vi "PID_controller_20.vi"() -> ()   [LabVIEW 2011]
panel:
  out "tFit_array":dbl[](array[numeric])
  out "PFit_array":dbl[](array[numeric])
  out "error array":dbl[](array[numeric])
  out "dt array":dbl[](array[numeric])
  out "Pset array":dbl[](array[numeric])
  out "t array":dbl[](array[numeric])
  out "P array":dbl[](array[numeric])
  in  "Local":bool
  in  "Hold":bool
  out "tune_Method":u16(ring) items=["Setpoint", "Angle"]
  in  "Method":u16(ring)=1 items=["Setpoint", "Angle"]
  in  "Setpoint":u16(ring)=2 items=["A", "B", "C", "D"]
  out "tuning":bool
  in  "Tune":bool
  out "Tune Set Point (torr)":dbl format="%.2f"
  in  "stop":bool
  out "err_avg":dbl
  out "Setpoint":string
  in  "Ks":dbl
  out "dt(s)":dbl
  out "windup error":dbl
  out "tPrev":dbl
  out "target value":dbl
  out "error":dbl
  out "tStart(s)":dbl
  out "S00":dbl
  out "S10":dbl
  out "S20":dbl
  out "S11":dbl
  out "S01":dbl
  out "weight array":dbl[](array[numeric])
  in  "# of points to watch":i32=60
  in  "tSmooth(s)":dbl=4.0
  out "IO error":errorcluster
  out "first":bool=TRUE
  out "XY Graph":cluster{"Value":dbl[], "Value":dbl[]}[](graph)
  out "current value":dbl
  in  "Period (s)":dbl=1.0
  out "dValue":dbl
  out "derivative":dbl
  out "integral":dbl
  in  "Angle (deg)":dbl format="%.1f"
  in  "Kd":dbl=0.4
  in  "Ki":dbl
  in  "Kp":dbl=0.1
  out "P (torr)":dbl format="%.2f"
  in  "Set Point (torr)":dbl format="%.2f"
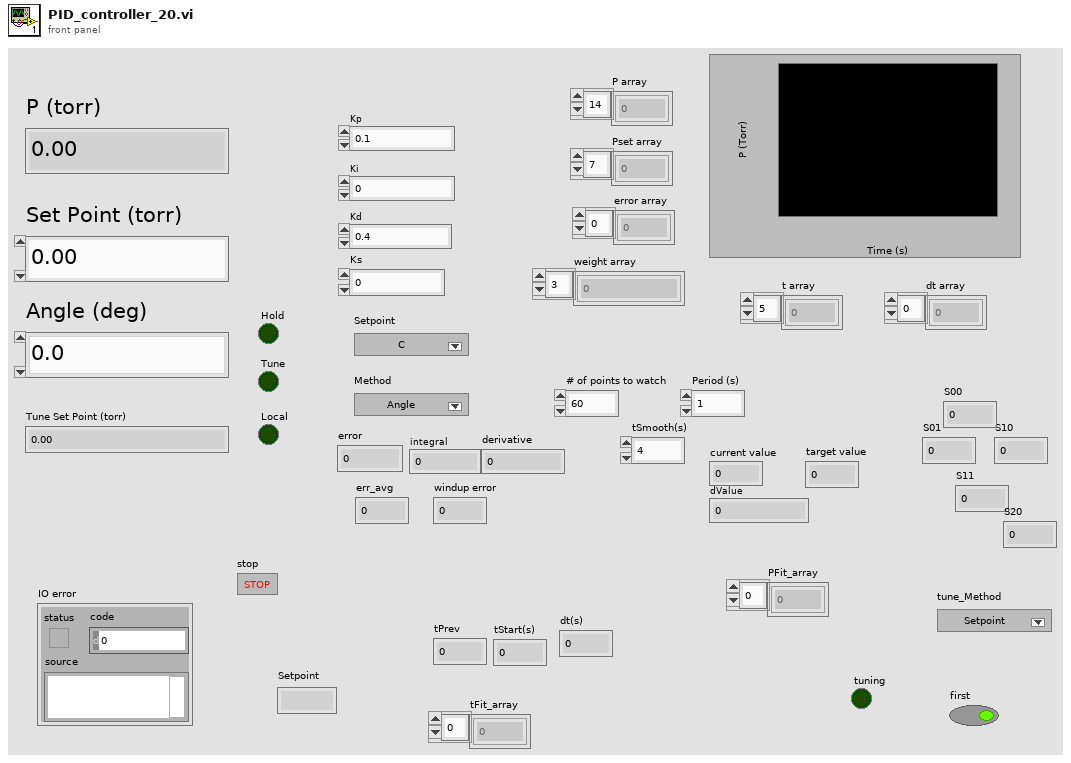
[diagram p1: front panel]
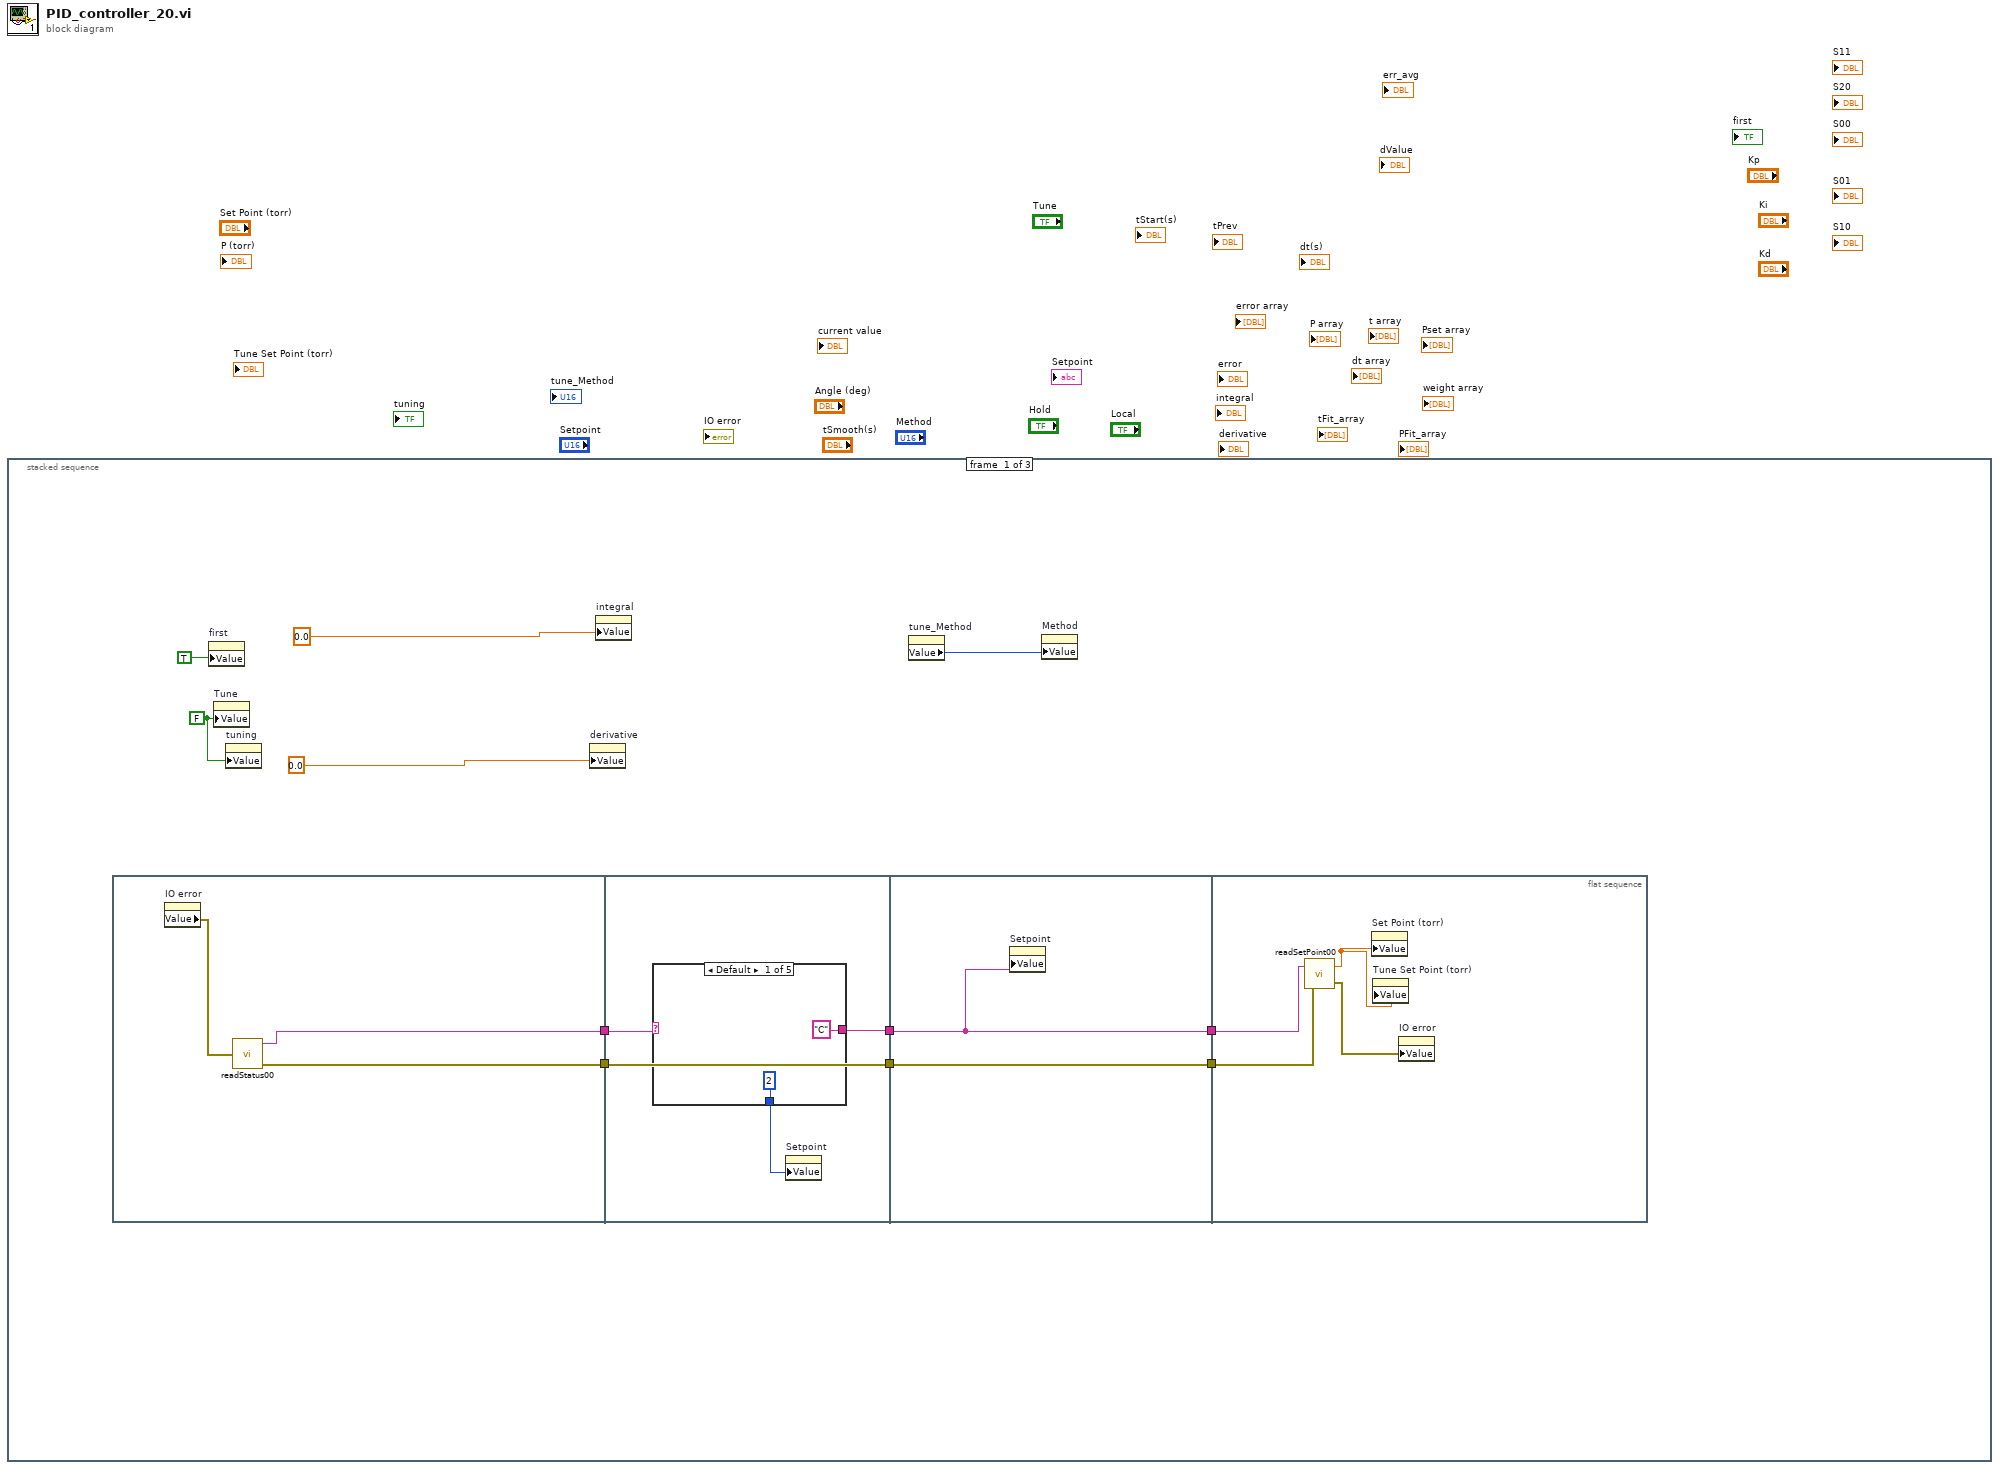
[diagram p0: block diagram]
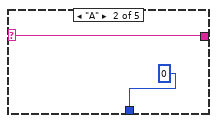
[diagram p2: hidden frame]
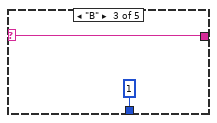
[diagram p3: hidden frame]
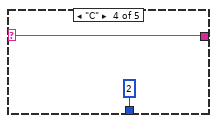
[diagram p4: hidden frame]
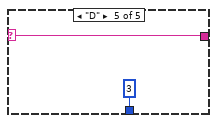
[diagram p5: hidden frame]
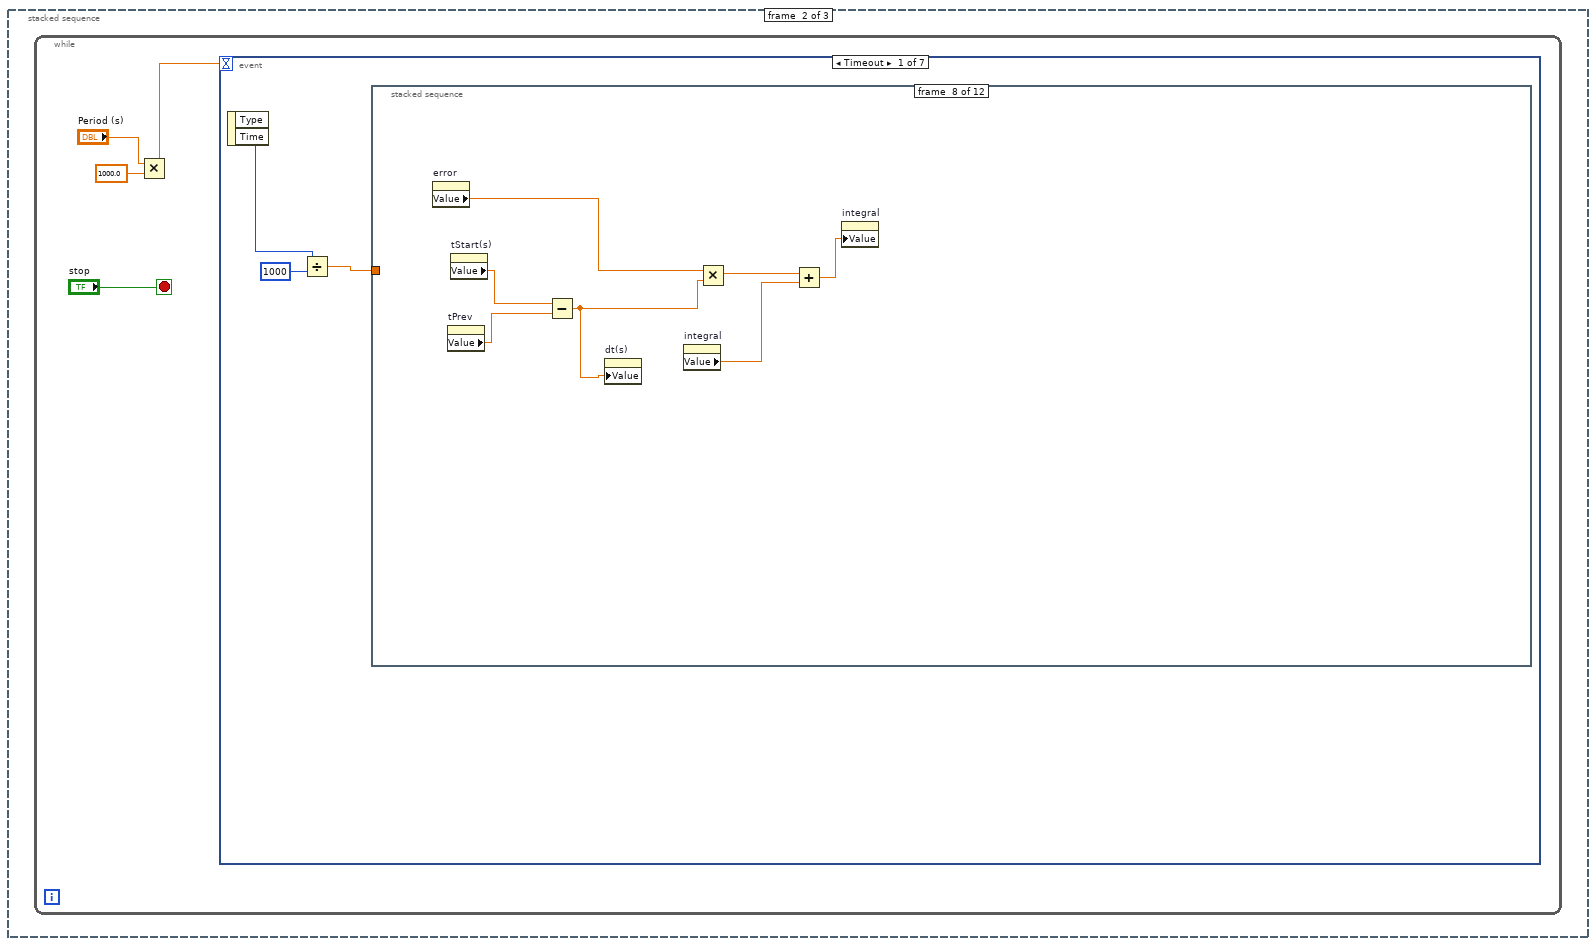
[diagram p6: hidden frame]
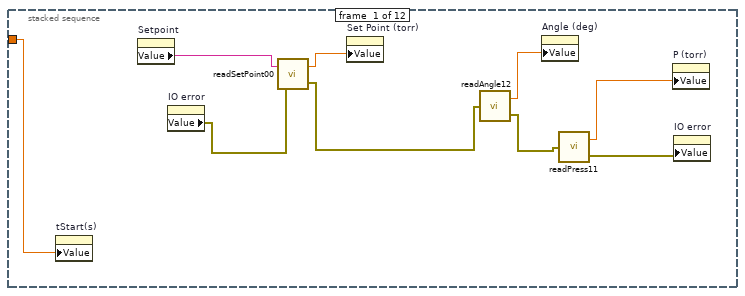
[diagram p7: hidden frame]
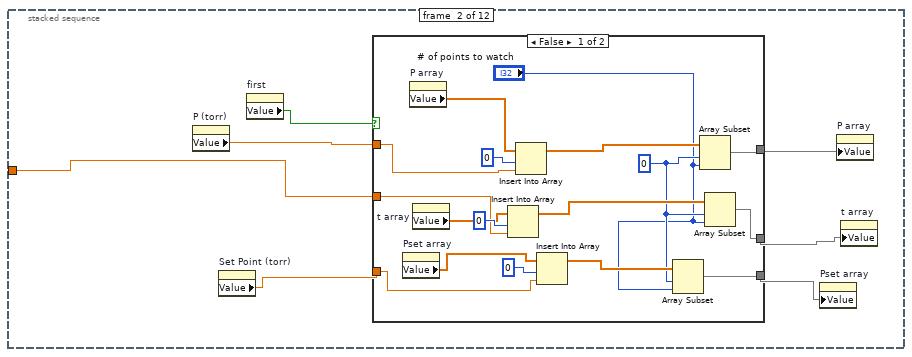
[diagram p8: hidden frame]
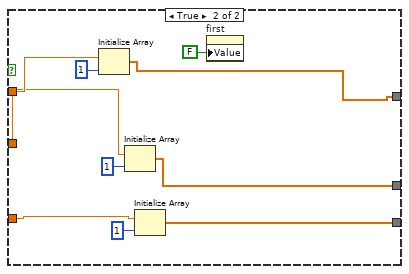
[diagram p9: hidden frame]
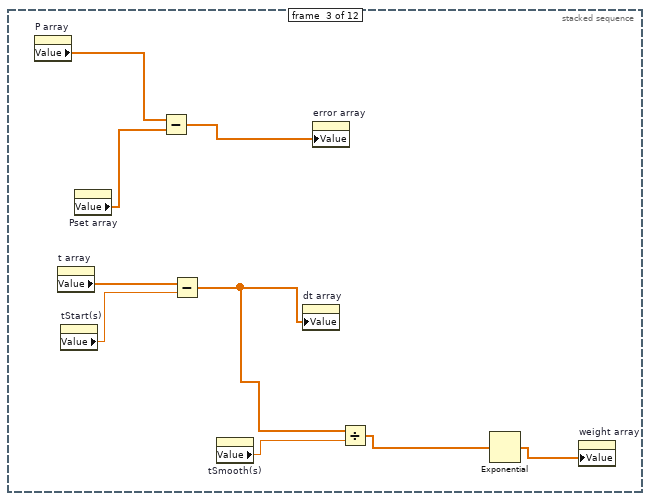
[diagram p10: hidden frame]
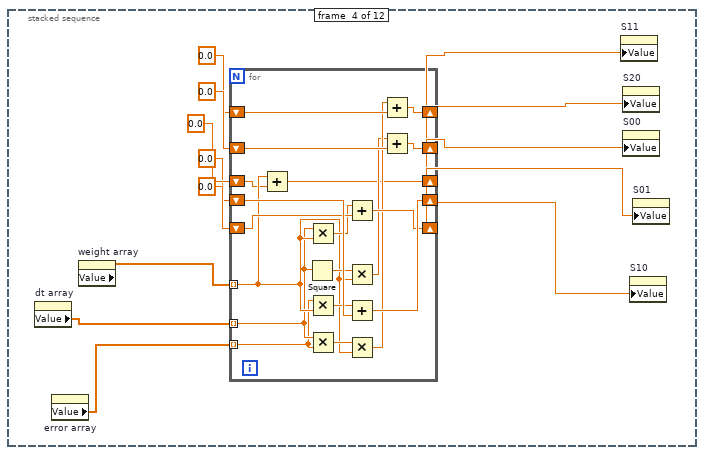
[diagram p11: hidden frame]
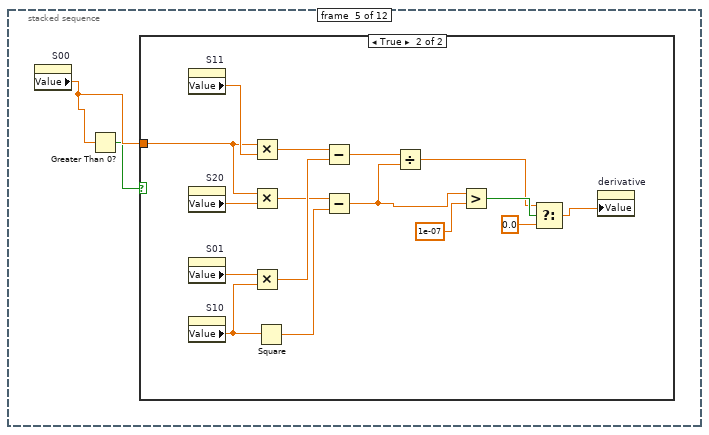
[diagram p12: hidden frame]
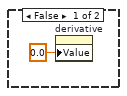
[diagram p13: hidden frame]
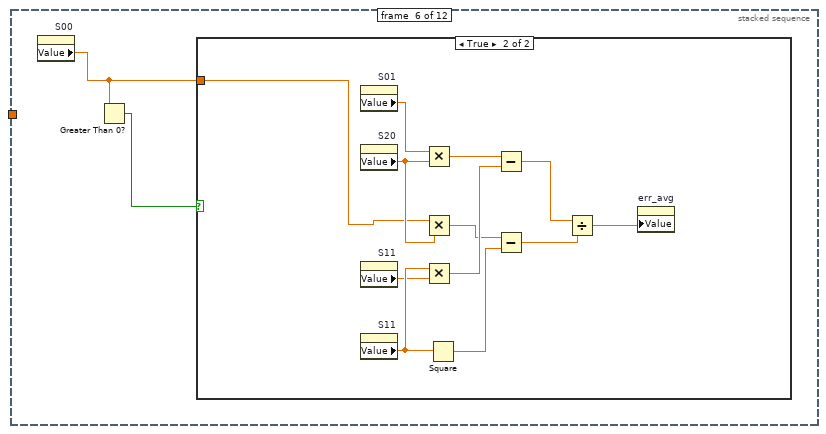
[diagram p14: hidden frame]
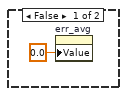
[diagram p15: hidden frame]
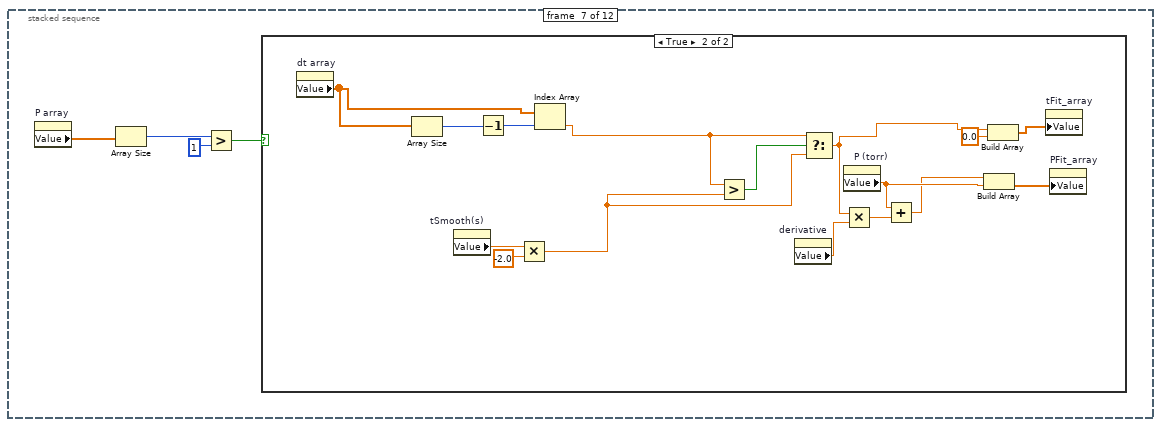
[diagram p16: hidden frame]
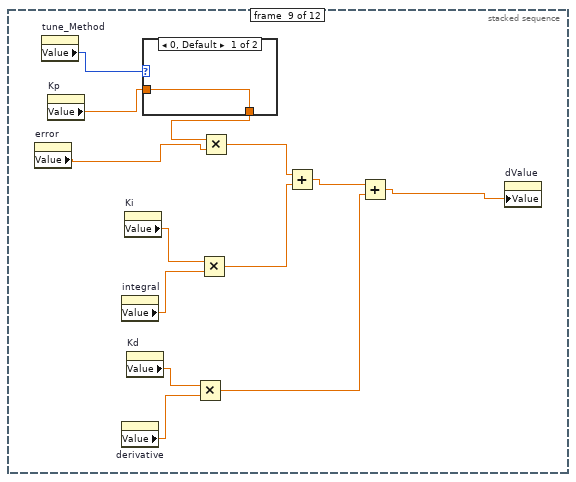
[diagram p18: hidden frame]
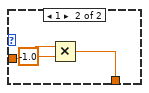
[diagram p19: hidden frame]
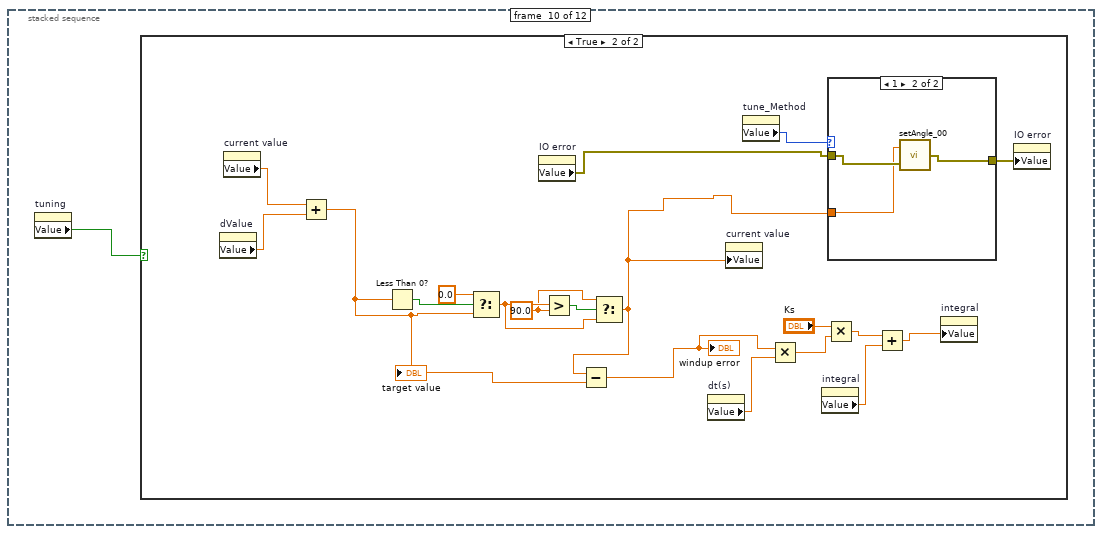
[diagram p20: hidden frame]
diagram:
  n1 = stacked-sequence {
    frame #0 {
      w8 = FALSE ("Tune")
      n2 = flat-sequence {
        tunnel: [w13] -> w7
        tunnel: [w12] -> w6
        tunnel: w7 -> [w17]
        tunnel: [w16] -> w5
        tunnel: w6 -> [w18]
        tunnel: [w18] -> w3
        tunnel: w5 -> [w29]
        tunnel: [w29] -> w4
        tunnel: w3 -> [w30]
        tunnel: [w30] -> w2
        tunnel: w4 -> [w34]
        tunnel: w2 -> [w33]
        frame #0 {
          n3 = property on="IO error" class="Clust (strict)"() -> ("Value"=w14:errorcluster)  [unwired: 2 in, 2 out]
          n4 = call "readStatus00.vi"("error in"=w14) -> ("Setpoint"=w13:string, "error out"=w12:errorcluster)  [unwired: 1 out]
        }
        frame #1 {
          n5 = case shown="Default" w17 {
            selector: w17 -> [_ w22 w23 w25 w27]
            tunnel: ["C" w22 w23 w25 w27] -> w16
            tunnel: [u16 2 ("Ring") u16 0 ("Ring") u16 1 ("Ring") u16 2 ("Ring") u16 3 ("Ring")] -> w15
            frame Default {
            }
            frame "A" {
            }
            frame "B" {
            }
            frame "C" {
            }
            frame "D" {
            }
          }
          n6 = property on="Setpoint" class="Ring (strict)"("Value"=w15) -> ()  [unwired: 2 in, 2 out]
        }
        frame #2 {
          n7 = property on="Setpoint" class="Str"("Value"=w29) -> ()  [unwired: 2 in, 2 out]
        }
        frame #3 {
          n8 = call "readSetPoint00.vi"("error in"=w33, "Setpoint"=w34) -> ("error out"=w32:errorcluster, "P"=w31:dbl)
          n9 = property on="Set Point (torr)" class="DigNum (strict)"("Value"=w31) -> ()  [unwired: 2 in, 2 out]
          n10 = property on="Tune Set Point (torr)" class="DigNum (strict)"("Value"=w31) -> ()  [unwired: 2 in, 2 out]
          n11 = property on="IO error" class="Clust (strict)"("Value"=w32) -> ()  [unwired: 2 in, 2 out]
        }
      }
      n12 = property on="first" class="Bool (strict)"("Value"=TRUE ("first")) -> ()  [unwired: 2 in, 2 out]
      n13 = property on="Tune" class="Bool (strict)"("Value"=w8) -> ()  [unwired: 2 in, 2 out]
      n14 = property on="tuning" class="Bool (strict)"("Value"=w8) -> ()  [unwired: 2 in, 2 out]
      n15 = property on="derivative" class="DigNum (strict)"("Value"=0.0 ("derivative")) -> ()  [unwired: 2 in, 2 out]
      n16 = property on="integral" class="DigNum (strict)"("Value"=0.0 ("integral")) -> ()  [unwired: 2 in, 2 out]
      n17 = property on="tune_Method" class="Ring (strict)"() -> ("Value"=w1:u16)  [unwired: 2 in, 2 out]
      n18 = property on="Method" class="Ring (strict)"("Value"=w1) -> ()  [unwired: 2 in, 2 out]
    }
    frame #1 {
      n19 = while {
        stop <- "stop" stop-if-true
        n20 = Multiply(x="Period (s)", y=1000.0) -> (x*y=w36:dbl)
        n21 = event shown="[0] Timeout" {
          selector: _ -> [_ _ _ _ _ _ _]
          dyn-events: _ -> [_ _ _ _ _ _ _]
          timeout: w36 -> [_ _ _ _ _ _ _]
          event Timeout {
            n22 = event-data() -> ("Time"=w41:u32)  [unwired: 1 in, 1 out]
            n23 = Divide(x=w41, y=u32 1000) -> (x/y=w39:dbl)
            n24 = stacked-sequence {
              tunnel: w39 -> [w45 w57 _ _ _ _ _ _ _ _ _ _]
              frame #0 {
                n25 = property on="tStart(s)" class="DigNum (strict)"("Value"=w45) -> ()  [unwired: 2 in, 2 out]
                n26 = property on="Setpoint" class="Str"() -> ("Value"=w48:string)  [unwired: 2 in, 2 out]
                n27 = property on="IO error" class="Clust (strict)"() -> ("Value"=w49:errorcluster)  [unwired: 2 in, 2 out]
                n28 = call "readSetPoint00.vi"("error in"=w49, "Setpoint"=w48) -> ("error out"=w47:errorcluster, "P"=w50:dbl)
                n29 = property on="Set Point (torr)" class="DigNum (strict)"("Value"=w50) -> ()  [unwired: 2 in, 2 out]
                n30 = call "readAngle12.vi"("error in"=w47) -> ("angle"=w46:dbl, "error out"=w44:errorcluster)
                n31 = property on="Angle (deg)" class="DigNum (strict)"("Value"=w46) -> ()  [unwired: 2 in, 2 out]
                n32 = call "readPress11.vi"("error in"=w44) -> ("P"=w42:dbl, "error out"=w43:errorcluster)
                n33 = property on="P (torr)" class="DigNum (strict)"("Value"=w42) -> ()  [unwired: 2 in, 2 out]
                n34 = property on="IO error" class="Clust (strict)"("Value"=w43) -> ()  [unwired: 2 in, 2 out]
              }
              frame #1 {
                n35 = property on="P (torr)" class="DigNum (strict)"() -> ("Value"=w55:dbl)  [unwired: 2 in, 2 out]
                n36 = property on="Set Point (torr)" class="DigNum (strict)"() -> ("Value"=w52:dbl)  [unwired: 2 in, 2 out]
                n37 = property on="first" class="Bool (strict)"() -> ("Value"=w56:bool)  [unwired: 2 in, 2 out]
                n38 = case shown="False" w56 {
                  tunnel: w55 -> [w73 w83]
                  tunnel: [w64 w81] -> w54
                  tunnel: w57 -> [w70 w79]
                  tunnel: [w62 w78] -> w53
                  tunnel: w52 -> [w66 w76]
                  tunnel: [w58 w75] -> w51
                  frame False {
                    w60 = 0 ("index")
                    n39 = property on="Pset array" class="Arr (strict)"() -> ("Value"=w67:dbl[])  [unwired: 2 in, 2 out]
                    n40 = property on="P array" class="Arr (strict)"() -> ("Value"=w72:dbl[])  [unwired: 2 in, 2 out]
                    n41 = property on="t array" class="Arr (strict)"() -> ("Value"=w69:dbl[])  [unwired: 2 in, 2 out]
                    n42 = Insert Into Array(array=w69, index=0, new element=w70) -> (w63:dbl[])
                    n43 = Insert Into Array(array=w72, index=0, new element=w73) -> (w65:dbl[])
                    n44 = Insert Into Array(array=w67, index=0, new element=w66) -> (w61:dbl[])
                    n45 = Array Subset(array=w61, index=w60, length="# of points to watch") -> (w58:dbl[])
                    n46 = Array Subset(array=w65, index=w60, length="# of points to watch") -> (w64:dbl[])
                    n47 = Array Subset(array=w63, index=w60, length="# of points to watch") -> (w62:dbl[])
                  }
                  frame True {
                    n48 = Initialize Array(w83, 1 ("dimension size")) -> (w81:dbl[])
                    n49 = Initialize Array(w79, 1 ("dimension size")) -> (w78:dbl[])
                    n50 = Initialize Array(w76, 1 ("dimension size")) -> (w75:dbl[])
                    n51 = property on="first" class="Bool (strict)"("Value"=FALSE ("first")) -> ()  [unwired: 2 in, 2 out]
                  }
                }
                n52 = property on="Pset array" class="Arr (strict)"("Value"=w51) -> ()  [unwired: 2 in, 2 out]
                n53 = property on="P array" class="Arr (strict)"("Value"=w54) -> ()  [unwired: 2 in, 2 out]
                n54 = property on="t array" class="Arr (strict)"("Value"=w53) -> ()  [unwired: 2 in, 2 out]
              }
              frame #2 {
                n55 = property on="P array" class="Arr (strict)"() -> ("Value"=w87:dbl[])  [unwired: 2 in, 2 out]
                n56 = property on="t array" class="Arr (strict)"() -> ("Value"=w93:dbl[])  [unwired: 2 in, 2 out]
                n57 = property on="tStart(s)" class="DigNum (strict)"() -> ("Value"=w92:dbl)  [unwired: 2 in, 2 out]
                n58 = property on="Pset array" class="Arr (strict)"() -> ("Value"=w86:dbl[])  [unwired: 2 in, 2 out]
                n59 = Subtract(x=w87, y=w86) -> (x-y=w85:dbl[])
                n60 = Subtract(x=w93, y=w92) -> (x-y=w89:dbl[])
                n61 = property on="tSmooth(s)" class="DigNum (strict)"() -> ("Value"=w91:dbl)  [unwired: 2 in, 2 out]
                n62 = property on="dt array" class="Arr (strict)"("Value"=w89) -> ()  [unwired: 2 in, 2 out]
                n63 = property on="error array" class="Arr (strict)"("Value"=w85) -> ()  [unwired: 2 in, 2 out]
                n64 = Divide(x=w89, y=w91) -> (x/y=w90:dbl[])
                n65 = Exponential(1:w90) -> (0:w88:dbl[])
                n66 = property on="weight array" class="Arr (strict)"("Value"=w88) -> ()  [unwired: 2 in, 2 out]
              }
              frame #3 {
                n67 = property on="dt array" class="Arr (strict)"() -> ("Value"=w95:dbl[])  [unwired: 2 in, 2 out]
                n68 = property on="error array" class="Arr (strict)"() -> ("Value"=w94:dbl[])  [unwired: 2 in, 2 out]
                n69 = property on="weight array" class="Arr (strict)"() -> ("Value"=w100:dbl[])  [unwired: 2 in, 2 out]
                n70 = for {
                  shift-right: [w122] -> w105
                  shift-left: 0.0 -> [w125]
                  shift-right: [w119] -> w102
                  shift-left: 0.0 -> [w124]
                  shift-right: [w118] -> w103
                  shift-left: 0.0 -> [w123]
                  shift-right: [w120] -> w106
                  shift-left: 0.0 -> [w121]
                  tunnel: w100 -> [w111] mode=indexing
                  shift-right: [w109] -> w104
                  shift-left: 0.0 -> [w110]
                  tunnel: w95 -> [w108] mode=indexing
                  tunnel: w94 -> [w107] mode=indexing
                  n71 = Add(x=w111, y=w110) -> (x+y=w109:dbl)
                  n72 = Square(x=w108) -> (x^2=w114:dbl)
                  n73 = Multiply(x=w108, y=w111) -> (x*y=w112:dbl)
                  n74 = Multiply(x=w107, y=w111) -> (x*y=w117:dbl)
                  n75 = Multiply(x=w108, y=w107) -> (x*y=w116:dbl)
                  n76 = Add(x=w112, y=w121) -> (x+y=w120:dbl)
                  n77 = Multiply(x=w114, y=w111) -> (x*y=w113:dbl)
                  n78 = Add(x=w117, y=w125) -> (x+y=w122:dbl)
                  n79 = Multiply(x=w116, y=w111) -> (x*y=w115:dbl)
                  n80 = Add(x=w115, y=w124) -> (x+y=w119:dbl)
                  n81 = Add(x=w113, y=w123) -> (x+y=w118:dbl)
                }
                n82 = property on="S11" class="DigNum (strict)"("Value"=w102) -> ()  [unwired: 2 in, 2 out]
                n83 = property on="S20" class="DigNum (strict)"("Value"=w103) -> ()  [unwired: 2 in, 2 out]
                n84 = property on="S00" class="DigNum (strict)"("Value"=w104) -> ()  [unwired: 2 in, 2 out]
                n85 = property on="S10" class="DigNum (strict)"("Value"=w106) -> ()  [unwired: 2 in, 2 out]
                n86 = property on="S01" class="DigNum (strict)"("Value"=w105) -> ()  [unwired: 2 in, 2 out]
              }
              frame #4 {
                n87 = property on="S00" class="DigNum (strict)"() -> ("Value"=w127:dbl)  [unwired: 2 in, 2 out]
                n88 = Greater Than 0?(x=w127) -> (x > 0?=w126:bool)
                n89 = case shown="True" w126 {
                  tunnel: w127 -> [_ w136]
                  frame False {
                    n90 = property on="derivative" class="DigNum (strict)"("Value"=0.0 ("derivative")) -> ()  [unwired: 2 in, 2 out]
                  }
                  frame True {
                    n91 = property on="S11" class="DigNum (strict)"() -> ("Value"=w138:dbl)  [unwired: 2 in, 2 out]
                    n92 = property on="S20" class="DigNum (strict)"() -> ("Value"=w137:dbl)  [unwired: 2 in, 2 out]
                    n93 = property on="S01" class="DigNum (strict)"() -> ("Value"=w135:dbl)  [unwired: 2 in, 2 out]
                    n94 = property on="S10" class="DigNum (strict)"() -> ("Value"=w139:dbl)  [unwired: 2 in, 2 out]
                    n95 = Multiply(x=w136, y=w138) -> (x*y=w144:dbl)
                    n96 = Multiply(x=w136, y=w137) -> (x*y=w142:dbl)
                    n97 = Multiply(x=w135, y=w139) -> (x*y=w143:dbl)
                    n98 = Square(x=w139) -> (x^2=w141:dbl)
                    n99 = Subtract(x=w144, y=w143) -> (x-y=w140:dbl)
                    n100 = Subtract(x=w142, y=w141) -> (x-y=w134:dbl)
                    n101 = Divide(x=w140, y=w134) -> (x/y=w130:dbl)
                    n102 = Greater?(x=w134, y=1e-07) -> (0:w132:bool)
                    n103 = Select(t=w130, s=w132, f=0.0) -> (s? t:f=w131:dbl)
                    n104 = property on="derivative" class="DigNum (strict)"("Value"=w131) -> ()  [unwired: 2 in, 2 out]
                  }
                }
              }
              frame #5 {
                n105 = property on="S00" class="DigNum (strict)"() -> ("Value"=w146:dbl)  [unwired: 2 in, 2 out]
                n106 = Greater Than 0?(x=w146) -> (x > 0?=w145:bool)
                n107 = case shown="True" w145 {
                  tunnel: w146 -> [_ w149]
                  frame False {
                    n108 = property on="err_avg" class="DigNum (strict)"("Value"=0.0 ("Pavg")) -> ()  [unwired: 2 in, 2 out]
                  }
                  frame True {
                    n109 = property on="S01" class="DigNum (strict)"() -> ("Value"=w150:dbl)  [unwired: 2 in, 2 out]
                    n110 = property on="S20" class="DigNum (strict)"() -> ("Value"=w153:dbl)  [unwired: 2 in, 2 out]
                    n111 = property on="S11" class="DigNum (strict)"() -> ("Value"=w151:dbl)  [unwired: 2 in, 2 out]
                    n112 = property on="S11" class="DigNum (strict)"() -> ("Value"=w152:dbl)  [unwired: 2 in, 2 out]
                    n113 = Multiply(x=w150, y=w153) -> (x*y=w158:dbl)
                    n114 = Multiply(x=w149, y=w153) -> (x*y=w155:dbl)
                    n115 = Multiply(x=w152, y=w151) -> (x*y=w159:dbl)
                    n116 = Square(x=w152) -> (x^2=w156:dbl)
                    n117 = Subtract(x=w158, y=w159) -> (x-y=w154:dbl)
                    n118 = Subtract(x=w155, y=w156) -> (x-y=w157:dbl)
                    n119 = Divide(x=w154, y=w157) -> (x/y=w148:dbl)
                    n120 = property on="err_avg" class="DigNum (strict)"("Value"=w148) -> ()  [unwired: 2 in, 2 out]
                  }
                }
              }
              frame #6 {
                n121 = property on="P array" class="Arr (strict)"() -> ("Value"=w160:dbl[])  [unwired: 2 in, 2 out]
                n122 = Array Size(array=w160) -> (size(s)=w161:i32)
                n123 = Greater?(x=w161, y=1) -> (0:w163:bool)
                n124 = case shown="True" w163 {
                  frame False {
                  }
                  frame True {
                    n125 = property on="dt array" class="Arr (strict)"() -> ("Value"=w171:dbl[])  [unwired: 2 in, 2 out]
                    n126 = Array Size(array=w171) -> (size(s)=w179:i32)
                    n127 = property on="tSmooth(s)" class="DigNum (strict)"() -> ("Value"=w173:dbl)  [unwired: 2 in, 2 out]
                    n128 = Decrement(x=w179) -> (x-1=w178:i32)
                    n129 = Multiply(x=w173, y=-2.0) -> (x*y=w164:dbl)
                    n130 = Index Array(array=w171, index=w178) -> (element=w172:dbl)
                    n131 = Greater?(x=w172, y=w164) -> (0:w175:bool)
                    n132 = property on="derivative" class="DigNum (strict)"() -> ("Value"=w177:dbl)  [unwired: 2 in, 2 out]
                    n133 = Select(t=w172, s=w175, f=w164) -> (s? t:f=w168:dbl)
                    n134 = property on="P (torr)" class="DigNum (strict)"() -> ("Value"=w170:dbl)  [unwired: 2 in, 2 out]
                    n135 = Multiply(x=w168, y=w177) -> (x*y=w176:dbl)
                    n136 = Add(x=w170, y=w176) -> (x+y=w169:dbl)
                    n137 = Build Array(w169, w170) -> (w165:dbl[])
                    n138 = Build Array(w168, 0.0 ("element")) -> (w166:dbl[])
                    n139 = property on="tFit_array" class="Arr (strict)"("Value"=w166) -> ()  [unwired: 2 in, 2 out]
                    n140 = property on="PFit_array" class="Arr (strict)"("Value"=w165) -> ()  [unwired: 2 in, 2 out]
                  }
                }
              }
              frame #7 {
                n141 = property on="error" class="DigNum (strict)"() -> ("Value"=w182:dbl)  [unwired: 2 in, 2 out]
                n142 = property on="tPrev" class="DigNum (strict)"() -> ("Value"=w181:dbl)  [unwired: 2 in, 2 out]
                n143 = property on="tStart(s)" class="DigNum (strict)"() -> ("Value"=w180:dbl)  [unwired: 2 in, 2 out]
                n144 = Subtract(x=w180, y=w181) -> (x-y=w186:dbl)
                n145 = property on="dt(s)" class="DigNum (strict)"("Value"=w186) -> ()  [unwired: 2 in, 2 out]
                n146 = property on="integral" class="DigNum (strict)"() -> ("Value"=w184:dbl)  [unwired: 2 in, 2 out]
                n147 = Multiply(x=w182, y=w186) -> (x*y=w183:dbl)
                n148 = Add(x=w183, y=w184) -> (x+y=w185:dbl)
                n149 = property on="integral" class="DigNum (strict)"("Value"=w185) -> ()  [unwired: 2 in, 2 out]
              }
              frame #8 {
                n150 = property on="error" class="DigNum (strict)"() -> ("Value"=w199:dbl)  [unwired: 2 in, 2 out]
                n151 = property on="tune_Method" class="Ring (strict)"() -> ("Value"=w189:u16)  [unwired: 2 in, 2 out]
                n152 = property on="Kp" class="DigNum (strict)"() -> ("Value"=w188:dbl)  [unwired: 2 in, 2 out]
                n153 = property on="integral" class="DigNum (strict)"() -> ("Value"=w191:dbl)  [unwired: 2 in, 2 out]
                n154 = property on="derivative" class="DigNum (strict)"() -> ("Value"=w193:dbl)  [unwired: 2 in, 2 out]
                n155 = property on="Ki" class="DigNum (strict)"() -> ("Value"=w190:dbl)  [unwired: 2 in, 2 out]
                n156 = property on="Kd" class="DigNum (strict)"() -> ("Value"=w192:dbl)  [unwired: 2 in, 2 out]
                n157 = case shown="0, Default" w189 {
                  tunnel: w188 -> [w200 w203]
                  tunnel: [w200 w201] -> w187
                  frame 0, Default {
                  }
                  frame 1 {
                    n158 = Multiply(x=w203, y=-1.0) -> (x*y=w201:dbl)
                  }
                }
                n159 = Multiply(x=w192, y=w193) -> (x*y=w196:dbl)
                n160 = Multiply(x=w190, y=w191) -> (x*y=w195:dbl)
                n161 = Multiply(x=w187, y=w199) -> (x*y=w194:dbl)
                n162 = Add(x=w194, y=w195) -> (x+y=w197:dbl)
                n163 = Add(x=w197, y=w196) -> (x+y=w198:dbl)
                n164 = property on="dValue" class="DigNum (strict)"("Value"=w198) -> ()  [unwired: 2 in, 2 out]
              }
              frame #9 {
                n165 = property on="tuning" class="Bool (strict)"() -> ("Value"=w204:bool)  [unwired: 2 in, 2 out]
                n166 = case shown="True" w204 {
                  frame False {
                  }
                  frame True {
                    w217 = 90.0 ("y")
                    n167 = property on="dValue" class="DigNum (strict)"() -> ("Value"=w222:dbl)  [unwired: 2 in, 2 out]
                    n168 = property on="current value" class="DigNum (strict)"() -> ("Value"=w223:dbl)  [unwired: 2 in, 2 out]
                    n169 = Add(x=w223, y=w222) -> (x+y=w209:dbl)
                    "target value" <- w209
                    n170 = Less Than 0?(x=w209) -> (x < 0?=w221:bool)
                    n171 = Select(t=0.0, s=w221, f=w209) -> (s? t:f=w218:dbl)
                    n172 = property on="IO error" class="Clust (strict)"() -> ("Value"=w207:errorcluster)  [unwired: 2 in, 2 out]
                    n173 = Greater?(x=w218, y=w217) -> (0:w219:bool)
                    n174 = Select(t=w217, s=w219, f=w218) -> (s? t:f=w206:dbl)
                    n175 = Subtract(x=w206, y=w209) -> (x-y=w216:dbl)
                    "windup error" <- w216
                    n176 = property on="dt(s)" class="DigNum (strict)"() -> ("Value"=w215:dbl)  [unwired: 2 in, 2 out]
                    n177 = property on="current value" class="DigNum (strict)"("Value"=w206) -> ()  [unwired: 2 in, 2 out]
                    n178 = property on="tune_Method" class="Ring (strict)"() -> ("Value"=w208:u16)  [unwired: 2 in, 2 out]
                    n179 = Multiply(x=w216, y=w215) -> (x*y=w214:dbl)
                    n180 = property on="integral" class="DigNum (strict)"() -> ("Value"=w211:dbl)  [unwired: 2 in, 2 out]
                    n181 = Multiply(x="Ks", y=w214) -> (x*y=w212:dbl)
                    n182 = case shown="1" w208 {
                      tunnel: w207 -> [w227 w230]
                      tunnel: w206 -> [w226 w229]
                      tunnel: [w224 w228] -> w205
                      frame 0, Default {
                        n183 = property on="Setpoint" class="Str"() -> ("Value"=w225:string)  [unwired: 2 in, 2 out]
                        n184 = property on="Tune Set Point (torr)" class="DigNum (strict)"("Value"=w226) -> ()  [unwired: 2 in, 2 out]
                        n185 = call "writeSetPoint_00.vi"("error in"=w227, "P (Torr)"=w226, "Setpoint"=w225) -> ("error out"=w224:errorcluster)
                      }
                      frame 1 {
                        n186 = call "setAngle_00.vi"("error in (no error)"=w230, "Angle (deg)"=w229) -> ("error out"=w228:errorcluster)
                      }
                    }
                    n187 = Add(x=w212, y=w211) -> (x+y=w210:dbl)
                    n188 = property on="integral" class="DigNum (strict)"("Value"=w210) -> ()  [unwired: 2 in, 2 out]
                    n189 = property on="IO error" class="Clust (strict)"("Value"=w205) -> ()  [unwired: 2 in, 2 out]
                  }
                }
              }
              frame #10 {
                n190 = property on="dt array" class="Arr (strict)"() -> ("Value"=w232:dbl[])  [unwired: 2 in, 2 out]
                n191 = property on="PFit_array" class="Arr (strict)"() -> ("Value"=w237:dbl[])  [unwired: 2 in, 2 out]
                n192 = property on="tFit_array" class="Arr (strict)"() -> ("Value"=w238:dbl[])  [unwired: 2 in, 2 out]
                n193 = property on="P array" class="Arr (strict)"() -> ("Value"=w239:dbl[])  [unwired: 2 in, 2 out]
                n194 = property on="Pset array" class="Arr (strict)"() -> ("Value"=w233:dbl[])  [unwired: 2 in, 2 out]
                n195 = Bundle("Value"=w232, "Value"=w233) -> (w231:cluster{"Value":dbl[], "Value":dbl[]})  [unwired: 1 in]
                n196 = Bundle("Value"=w238, "Value"=w237) -> (w235:cluster{"Value":dbl[], "Value":dbl[]})  [unwired: 1 in]
                n197 = Bundle("Value"=w232, "Value"=w239) -> (w236:cluster{"Value":dbl[], "Value":dbl[]})  [unwired: 1 in]
                n198 = Build Array(w236, w235, w231) -> (→"XY Graph":cluster{"Value":dbl[], "Value":dbl[]}[])
              }
              frame #11 {
                n199 = property on="tStart(s)" class="DigNum (strict)"() -> ("Value"=w240:dbl)  [unwired: 2 in, 2 out]
                n200 = property on="tPrev" class="DigNum (strict)"("Value"=w240) -> ()  [unwired: 2 in, 2 out]
              }
            }
          }
          event "Hold": Value Change {
            n201 = event-data() -> ()  [unwired: 1 in, 5 out]
            n202 = property on="Hold" class="Bool (strict)"() -> ("Value"=w241:bool)  [unwired: 2 in, 2 out]
            n203 = case shown="False" w241 {
              frame False {
                n204 = property on="Local" class="Bool (strict)"() -> ("Value"=w242:bool)  [unwired: 2 in, 2 out]
                n205 = case shown="False" w242 {
                  frame False {
                    n206 = property on="IO error" class="Clust (strict)"() -> ("Value"=w246:errorcluster)  [unwired: 2 in, 2 out]
                    n207 = property on="Setpoint" class="Str"() -> ("Value"=w243:string)  [unwired: 2 in, 2 out]
                    n208 = call "readSetPoint00.vi"("error in"=w246, "Setpoint"=w243) -> ("error out"=w245:errorcluster, "P"=w244:dbl)
                    n209 = property on="Tune Set Point (torr)" class="DigNum (strict)"("Value"=w244) -> ()  [unwired: 2 in, 2 out]
                    n210 = property on="Set Point (torr)" class="DigNum (strict)"("Value"=w244) -> ()  [unwired: 2 in, 2 out]
                    n211 = property on="IO error" class="Clust (strict)"("Value"=w245) -> ()  [unwired: 2 in, 2 out]
                  }
                  frame True {
                  }
                }
              }
              frame True {
                n212 = property on="IO error" class="Clust (strict)"() -> ("Value"=w250:errorcluster)  [unwired: 2 in, 2 out]
                n213 = property on="Tune" class="Bool (strict)"("Value"=FALSE ("Tune")) -> ()  [unwired: 2 in, 2 out]
                n214 = property on="Local" class="Bool (strict)"("Value"=FALSE ("Local")) -> ()  [unwired: 2 in, 2 out]
                n215 = call "WriteAdaptorr03.vi"("error in (no error)"=w250, "string to write"="H") -> ("error out"=w249:errorcluster)
                n216 = property on="IO error" class="Clust (strict)"("Value"=w249) -> ()  [unwired: 2 in, 2 out]
              }
            }
          }
          event "Local": Value Change {
            n217 = event-data() -> ()  [unwired: 1 in, 5 out]
            n218 = property on="Local" class="Bool (strict)"() -> ("Value"=w252:bool)  [unwired: 2 in, 2 out]
            n219 = case shown="True" w252 {
              frame False {
                n220 = property on="IO error" class="Clust (strict)"() -> ("Value"=w255:errorcluster)  [unwired: 2 in, 2 out]
                n221 = call "WriteAdaptorr03.vi"("error in (no error)"=w255, "string to write"="H") -> ("error out"=w254:errorcluster)
                n222 = property on="Hold" class="Bool (strict)"("Value"=TRUE ("Hold")) -> ()  [unwired: 2 in, 2 out]
                n223 = property on="IO error" class="Clust (strict)"("Value"=w254) -> ()  [unwired: 2 in, 2 out]
              }
              frame True {
                n224 = property on="IO error" class="Clust (strict)"() -> ("Value"=w259:errorcluster)  [unwired: 2 in, 2 out]
                n225 = call "WriteAdaptorr03.vi"("error in (no error)"=w259, "string to write"="D5") -> ("error out"=w260:errorcluster)
                n226 = property on="Hold" class="Bool (strict)"("Value"=FALSE ("Hold")) -> ()  [unwired: 2 in, 2 out]
                n227 = property on="IO error" class="Clust (strict)"("Value"=w260) -> ()  [unwired: 2 in, 2 out]
              }
            }
          }
          event "Tune": Value Change {
            n228 = event-data() -> ()  [unwired: 1 in, 5 out]
            n229 = property on="Tune" class="Bool (strict)"() -> ("Value"=w261:bool)  [unwired: 2 in, 2 out]
            n230 = property on="tuning" class="Bool (strict)"("Value"=w261) -> ()  [unwired: 2 in, 2 out]
            n231 = case shown="True" w261 {
              frame False {
                n232 = property on="tune_Method" class="Ring (strict)"() -> ("Value"=w262:u16)  [unwired: 2 in, 2 out]
                n233 = case shown="1" w262 {
                  frame 0, Default {
                    n234 = property on="Set Point (torr)" class="DigNum (strict)"() -> ("Value"=w265:dbl)  [unwired: 2 in, 2 out]
                    n235 = property on="Setpoint" class="Str"() -> ("Value"=w266:string)  [unwired: 2 in, 2 out]
                    n236 = property on="IO error" class="Clust (strict)"() -> ("Value"=w264:errorcluster)  [unwired: 2 in, 2 out]
                    n237 = call "writeSetPoint_00.vi"("error in"=w264, "P (Torr)"=w265, "Setpoint"=w266) -> ("error out"=w263:errorcluster)
                    n238 = property on="IO error" class="Clust (strict)"("Value"=w263) -> ()  [unwired: 2 in, 2 out]
                  }
                  frame 1 {
                    n239 = flat-sequence {
                      frame #0 {
                        n240 = call "WriteAdaptorr03.vi"("string to write"="D5") -> ()  [unwired: 1 in, 1 out]
                      }
                      frame #1 {
                        n241 = property on="Setpoint" class="Str"() -> ("Value"=w269:string)  [unwired: 2 in, 2 out]
                        n242 = Concatenate Strings("Press ", w269, " on AdapTorr") -> (w268:string)
                        n243 = One Button Dialog(message=w268) -> ()  [unwired: 1 in, 1 out]
                      }
                    }
                  }
                }
              }
              frame True {
                n244 = property on="tune_Method" class="Ring (strict)"() -> ("Value"=w273:u16)  [unwired: 2 in, 2 out]
                n245 = case shown="0, Default" w273 {
                  frame 0, Default {
                    n246 = property on="IO error" class="Clust (strict)"() -> ("Value"=w276:errorcluster)  [unwired: 2 in, 2 out]
                    n247 = property on="Setpoint" class="Str"() -> ("Value"=w275:string)  [unwired: 2 in, 2 out]
                    n248 = call "readSetPoint00.vi"("error in"=w276, "Setpoint"=w275) -> ("error out"=w277:errorcluster, "P"=w274:dbl)
                    n249 = property on="Tune Set Point (torr)" class="DigNum (strict)"("Value"=w274) -> ()  [unwired: 2 in, 2 out]
                    n250 = property on="Set Point (torr)" class="DigNum (strict)"("Value"=w274) -> ()  [unwired: 2 in, 2 out]
                    n251 = property on="IO error" class="Clust (strict)"("Value"=w277) -> ()  [unwired: 2 in, 2 out]
                    n252 = property on="current value" class="DigNum (strict)"("Value"=w274) -> ()  [unwired: 2 in, 2 out]
                  }
                  frame 1 {
                    n253 = property on="Angle (deg)" class="DigNum (strict)"() -> ("Value"=w278:dbl)  [unwired: 2 in, 2 out]
                    n254 = property on="current value" class="DigNum (strict)"("Value"=w278) -> ()  [unwired: 2 in, 2 out]
                  }
                }
                n255 = property on="integral" class="DigNum (strict)"("Value"=0.0 ("integral")) -> ()  [unwired: 2 in, 2 out]
              }
            }
          }
          event "Set Point (torr)": Value Change {
            n256 = event-data() -> ()  [unwired: 1 in, 5 out]
            n257 = property on="Set Point (torr)" class="DigNum (strict)"() -> ("Value"=w281:dbl)  [unwired: 2 in, 2 out]
            n258 = property on="Setpoint" class="Str"() -> ("Value"=w282:string)  [unwired: 2 in, 2 out]
            n259 = property on="IO error" class="Clust (strict)"() -> ("Value"=w280:errorcluster)  [unwired: 2 in, 2 out]
            n260 = call "writeSetPoint_00.vi"("error in"=w280, "P (Torr)"=w281, "Setpoint"=w282) -> ("error out"=w279:errorcluster)
            n261 = property on="IO error" class="Clust (strict)"("Value"=w279) -> ()  [unwired: 2 in, 2 out]
          }
          event "Setpoint": Value Change {
            n262 = event-data() -> ()  [unwired: 1 in, 5 out]
            n263 = property on="Setpoint" class="Ring (strict)"() -> ("Value"=w287:u16)  [unwired: 2 in, 2 out]
            n264 = case shown="3" w287 {
              tunnel: ["A" "B" "C" "D"] -> w283
              frame 0, Default {
              }
              frame 1 {
              }
              frame 2 {
              }
              frame 3 {
              }
            }
            n265 = property on="Setpoint" class="Str"("Value"=w283) -> ()  [unwired: 2 in, 2 out]
            n266 = property on="IO error" class="Clust (strict)"() -> ("Value"=w284:errorcluster)  [unwired: 2 in, 2 out]
            n267 = call "readSetPoint00.vi"("error in"=w284, "Setpoint"=w283) -> ("error out"=w285:errorcluster, "P"=w286:dbl)
            n268 = property on="Set Point (torr)" class="DigNum (strict)"("Value"=w286) -> ()  [unwired: 2 in, 2 out]
            n269 = property on="Tune Set Point (torr)" class="DigNum (strict)"("Value"=w286) -> ()  [unwired: 2 in, 2 out]
            n270 = property on="IO error" class="Clust (strict)"("Value"=w285) -> ()  [unwired: 2 in, 2 out]
          }
          event "Method": Value Change {
            n271 = event-data() -> ()  [unwired: 1 in, 5 out]
            n272 = property on="Method" class="Ring (strict)"() -> ("Value"=w292:u16)  [unwired: 2 in, 2 out]
            n273 = case shown="1" w292 {
              frame 0, Default {
              }
              frame 1 {
                n274 = property on="tuning" class="Bool (strict)"() -> ("Value"=w293:bool)  [unwired: 2 in, 2 out]
                n275 = case shown="True" w293 {
                  frame False {
                  }
                  frame True {
                    n276 = flat-sequence {
                      frame #0 {
                        n277 = call "WriteAdaptorr03.vi"("string to write"="D5") -> ()  [unwired: 1 in, 1 out]
                      }
                      frame #1 {
                        n278 = property on="Setpoint" class="Str"() -> ("Value"=w296:string)  [unwired: 2 in, 2 out]
                        n279 = Concatenate Strings("Press ", w296, " on AdapTorr") -> (w295:string)
                        n280 = One Button Dialog(message=w295) -> ()  [unwired: 1 in, 1 out]
                      }
                    }
                  }
                }
              }
            }
            n281 = property on="tune_Method" class="Ring (strict)"("Value"=w292) -> ()  [unwired: 2 in, 2 out]
          }
        }
      }
    }
    frame #2 {
      n282 = property on="tuning" class="Bool (strict)"() -> ("Value"=w299:bool)  [unwired: 2 in, 2 out]
      n283 = case shown="True" w299 {
        frame False {
        }
        frame True {
          n284 = property on="tune_Method" class="Ring (strict)"() -> ("Value"=w300:u16)  [unwired: 2 in, 2 out]
          n285 = case shown="1" w300 {
            frame 0, Default {
            }
            frame 1 {
              n286 = flat-sequence {
                frame #0 {
                  n287 = property on="IO error" class="Clust (strict)"() -> ("Value"=w302:errorcluster)  [unwired: 2 in, 2 out]
                  n288 = call "setLocal_And_Hold_00.vi"("error in (no error)"=w302) -> ("error out"=w301:errorcluster)
                  n289 = property on="IO error" class="Clust (strict)"("Value"=w301) -> ()  [unwired: 2 in, 2 out]
                }
                frame #1 {
                  n290 = property on="Setpoint" class="Str"() -> ("Value"=w304:string)  [unwired: 2 in, 2 out]
                  n291 = Concatenate Strings("Press ", w304, " on AdapTorr") -> (w303:string)
                  n292 = One Button Dialog(message=w303) -> ()  [unwired: 1 in, 1 out]
                }
              }
            }
          }
        }
      }
    }
  }
